vi "Fit Child VIs To Subpanel.vi"(8 "error in":errorcluster, 9 "scale VI layouts? (F)":bool, 10 "subpanel tag":string, 11 "state in":T1) -> (0 "error out":errorcluster, 3 "state out":T1)   [LabVIEW 2010, in "NI_SE_Config Front Panel Layout.lvlib"]
uses:
  NI_SE_Config Front Panel Layout.lvlib
  State.ctl
  VI Info.ctl
  VI Panel Layout/VI Panel Layout.lvclass
  Scaling Type.ctl
  Scaling Settings.ctl
  VI Panel Layout/VI Panel Layout.lvclass/VI Panel Layout.ctl
  VI Panel Layout/Get Subpanel VIs.vi
  NI_SE_Front Panel Layout.lvlib
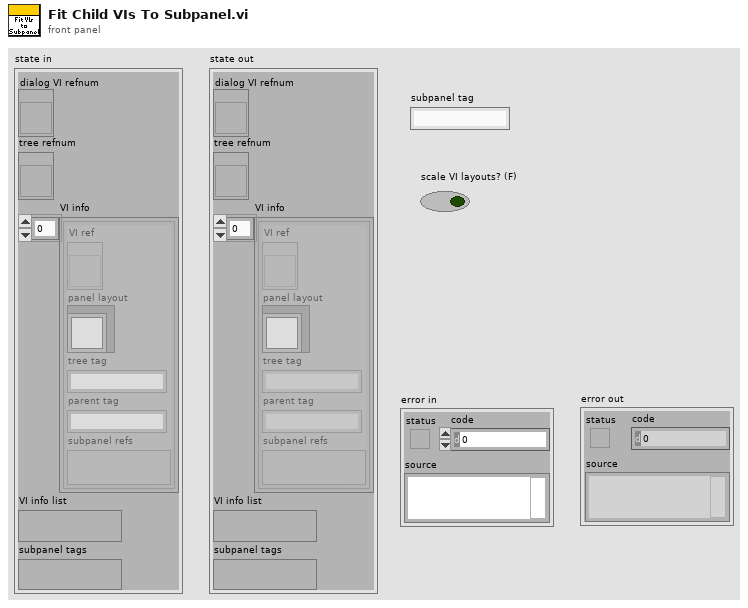
[diagram p1: front panel]
types:
  T1 = typedef "NI_SE_Config Front Panel Layout.lvlib/State.ctl" = cluster{"dialog VI refnum":refnum<vi>, "tree refnum":refnum<vi>, "VI info":T2[], "VI info list":variant, "subpanel tags":variant}
  T2 = typedef "NI_SE_Config Front Panel Layout.lvlib/VI Info.ctl" = cluster{"VI ref":refnum<vi>, "panel layout":refnum<class "VI Panel Layout.lvclass">, "tree tag":string, "parent tag":string, "subpanel refs":variant}
  T3 = typedef "NI_SE_Front Panel Layout.lvlib/Scaling Type.ctl" = enum16{"None", "Scale panel to fit layout", "Scale layout to fit panel"}
  T4 = typedef "NI_SE_Front Panel Layout.lvlib/Scaling Settings.ctl" = cluster{"scaling type":T3, "scale text":bool}
  T5 = typedef "LVBoundsTypeDef.ctl" = cluster{"Width":u32, "Height":u32}
  T6 = typedef "LVRectTypeDef.ctl" = cluster{"Left":i16, "Top":i16, "Right":i16, "Bottom":i16}
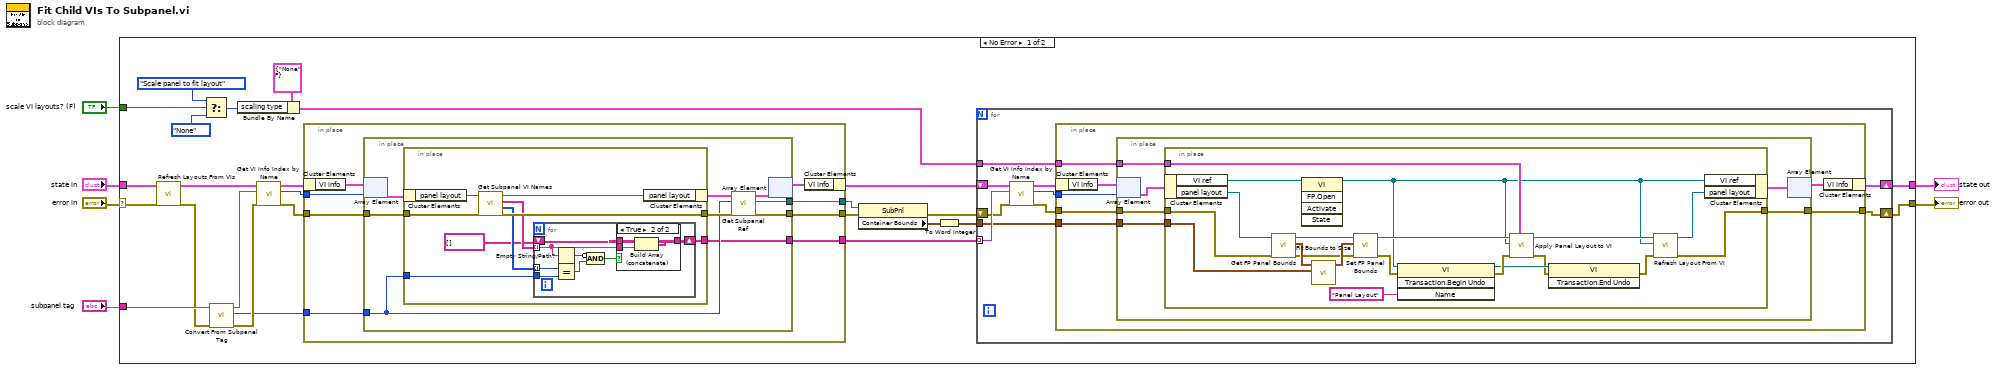
[diagram p0: block diagram]
diagram:
  n1 = case shown="No Error" "error in" {
    selector: "error in" -> [w15 w114]
    tunnel: "state in" -> [w17 w115]
    tunnel: [w19 w115] -> w4
    tunnel: [w18 w114] -> w3
    tunnel: "subpanel tag" -> [w32 _]
    tunnel: "scale VI layouts? (F)" -> [w10 _]
    frame No Error {
      n2 = call "Refresh Layouts From VIs.vi"("error in"=w15, "state in"=w17) -> ("error out"=w14:errorcluster, "state out"=w16:T1)  [unwired: 8 in]
      n3 = Select(t=Scaling_Type."Scale panel to fit layout" ("scaling type"), s=w10, f=Scaling_Type."None") -> (s? t:f=w8:T3)
      n4 = call "Convert From Subpanel Tag.vi"("error in"=w14, "subpanel tag"=w32) -> ("error out"=w30:errorcluster, "subpanel UID"=w26:i32, "owning VI name"=w31:string)  [unwired: 6 in, 1 out]
      n5 = Bundle By Name(cluster=T4 {"scaling type"=enum."None", "scale text"=FALSE} ("scaling settings"), "scaling type"=w8) -> (w11:T4)
      n6 = call "Get VI Info Index by Name.vi"("error in"=w30, "VI name"=w31, "state in"=w16) -> ("error out"=w28:errorcluster, "VI info index"=w27:i32, "state out"=w29:T1)  [unwired: 5 in, 1 out]
      n7 = in-place {
        in-place-border: w28 -> [w80]
        in-place-border: w27 -> [w82]
        in-place-border: w26 -> [w79]
        in-place-border: [w78] -> w24
        in-place-border: [w77] -> w25
        in-place-border: [w76] -> w22
        n8 = in-place-cluster #1(w29) -> ("VI info"=w83:T2[])
        n9 = in-place {
          in-place-border: w80 -> [w91]
          in-place-border: w79 -> [w86]
          in-place-border: [w88] -> w78
          in-place-border: [w85] -> w77
          in-place-border: [w84] -> w76
          n10 = in-place-array #2(w83, w82) -> (w92:T2)
          n11 = in-place {
            in-place-border: w91 -> [w99]
            in-place-border: w86 -> [w96]
            in-place-border: [w98] -> w87
            in-place-border: [w94] -> w84
            n12 = in-place-cluster #3(w92) -> ("panel layout"=w101:refnum<class "VI Panel Layout.lvclass">)
            n13 = call "Get Subpanel VI Names.vi"("error in (no error)"=w99, "VI Panel Layout in"=w101) -> ("error out"=w98:errorcluster, "subpanel object UIDs"=w97:i32[], "VI names"=w95:string[], "VI Panel Layout out"=w100:refnum<class "VI Panel Layout.lvclass">)  [unwired: 5 in, 1 out]
            n14 = for {
              tunnel: w97 -> [w109] mode=indexing
              tunnel: w96 -> [w108]
              tunnel: w95 -> [w107] mode=indexing
              shift-right: [w102] -> w94
              shift-left: string[] [] ("Array") -> [w103]
              n15 = Empty String/Path?(string/path=w107) -> (empty?=w106:bool)
              n16 = Equal?(x=w109, y=w108) -> (x = y?=w105:bool)
              n17 = Compound Arithmetic op=AND(invert w106, w105) -> (w104:bool)
              n18 = case shown="True" w104 {
                tunnel: w103 -> [w110 w112]
                tunnel: w107 -> [_ w111]
                tunnel: [w110 w113] -> w102
                frame False {
                }
                frame True {
                  n19 = Build Array (concatenate)(w112, w111) -> (w113:string[])
                }
              }
            }
            n20 = in-place-cluster #3("panel layout"=w100) -> (w90:T2)
          }
          n21 = call "Get Subpanel Ref.vi"("error in"=w87, "subpanel UID"=w86, "VI info in"=w90) -> ("error out"=w88:errorcluster, "subpanel ref"=w85:refnum<vi>, "VI info out"=w89:T2)  [unwired: 5 in, 1 out]
          n22 = in-place-array #2(w89) -> (w81:T2[])  [unwired: 1 out]
        }
        n23 = in-place-cluster #1("VI info"=w81) -> (w23:T1)
      }
      n24 = property class="SubPnl"(reference=w25, error in=w24) -> (error out=w21:errorcluster, "Container Bounds"=w20:T5)  [unwired: 1 out]
      n25 = To Word Integer(number=w20) -> (16bit integer=w13:cluster{"Width":i16, "Height":i16})
      n26 = for {
        shift-right: [w35] -> w19
        shift-left: w23 -> [w39]
        tunnel: w22 -> [w38] mode=indexing
        shift-right: [w33] -> w18
        shift-left: w21 -> [w37]
        tunnel: w13 -> [w36]
        tunnel: w11 -> [w34]
        n27 = call "Get VI Info Index by Name.vi"("error in"=w37, "VI name"=w38, "state in"=w39) -> ("error out"=w41:errorcluster, "VI info index"=w42:i32, "state out"=w40:T1)  [unwired: 5 in, 1 out]
        n28 = in-place {
          in-place-border: w41 -> [w46]
          in-place-border: w42 -> [w48]
          in-place-border: w36 -> [w45]
          in-place-border: w34 -> [w44]
          in-place-border: [w43] -> w33
          n29 = in-place-cluster #4(w40) -> ("VI info"=w49:T2[])
          n30 = in-place {
            in-place-border: w46 -> [w54]
            in-place-border: w45 -> [w53]
            in-place-border: w44 -> [w51]
            in-place-border: [w50] -> w43
            n31 = in-place-array #5(w49, w48) -> (w55:T2)
            n32 = in-place {
              in-place-border: w54 -> [w75]
              in-place-border: w53 -> [w73]
              in-place-border: w51 -> [w64]
              in-place-border: [w71] -> w50
              n33 = in-place-cluster #6(w55) -> ("VI ref"=w63:refnum<vi>, "panel layout"=w74:refnum<class "VI Panel Layout.lvclass">)
              n34 = call "Get FP Panel Bounds.vi"("error in (no error)"=w75, "VI Panel Layout in"=w74) -> ("error out"=w65:errorcluster, "FP panel bounds"=w68:T6, "VI Panel Layout out"=w67:refnum<class "VI Panel Layout.lvclass">)  [unwired: 7 in]
              n35 = invoke class="VI" method="FP.Open"(reference=w63) -> (reference out=w56:refnum<vi>)  [unwired: 4 in, 4 out]
              n36 = call "Fit Bounds to Size.vi"("size"=w73, "FP window bounds in"=w68) -> ("FP window bounds out"=w66:T6)  [unwired: 9 in]
              n37 = call "Set FP Panel Bounds.vi"("error in (no error)"=w65, "FP panel bounds"=w66, "VI Panel Layout in"=w67) -> ("error out"=w62:errorcluster, "VI Panel Layout out"=w70:refnum<class "VI Panel Layout.lvclass">)  [unwired: 7 in]
              n38 = invoke class="VI" method="Transaction.Begin Undo"(reference=w56, error in=w62, "Name"="Panel Layout") -> (reference out=w59:refnum<vi>, error out=w61:errorcluster)  [unwired: 1 in, 2 out]
              n39 = call "Apply Panel Layout to VI.vi"("scaling settings"=w64, "error in"=w61, "VI refnum"=w56, "panel layout in"=w70) -> ("error out"=w58:errorcluster, "panel layout out"=w72:refnum<class "VI Panel Layout.lvclass">)  [unwired: 6 in]
              n40 = invoke class="VI" method="Transaction.End Undo"(reference=w59, error in=w58) -> (error out=w57:errorcluster)  [unwired: 1 in, 2 out]
              n41 = call "Refresh Layout From VI.vi"("error in (no error)"=w57, "VI refnum"=w56, "VI Panel Layout in"=w72) -> ("error out"=w71:errorcluster, "VI Panel Layout out"=w69:refnum<class "VI Panel Layout.lvclass">)  [unwired: 5 in, 2 out]
              n42 = in-place-cluster #6("VI ref"=w56, "panel layout"=w69) -> (w52:T2)
            }
            n43 = in-place-array #5(w52) -> (w47:T2[])  [unwired: 1 out]
          }
          n44 = in-place-cluster #4("VI info"=w47) -> (w35:T1)
        }
      }
    }
    frame Error {
    }
  }
  "state out" <- w4
  "error out" <- w3
